vi "WebDAV address (global).vi"(0 "Network Drive IP":string, 1 "Mode":enum16{"Read", "Write"}(ring)) -> (2 "WebDAV Address":string)   [LabVIEW 2013]
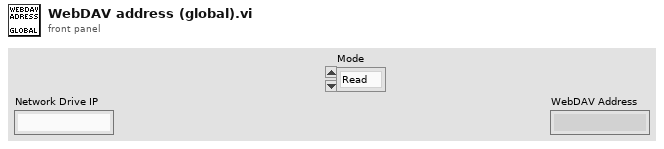
[diagram p1: front panel]
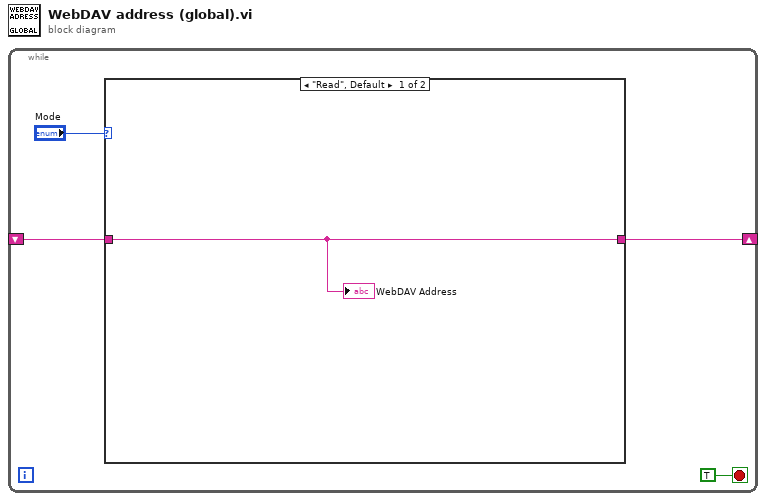
[diagram p0: block diagram]
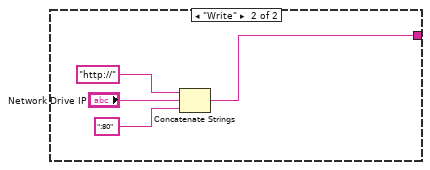
[diagram p2: hidden frame]
diagram:
  n1 = while {
    shift-right: [w2] -> _
    shift-left: _ -> [w1]
    stop <- TRUE stop-if-true
    n2 = case shown="\"Read\", Default" "Mode" {
      tunnel: [w5 w6] -> w2
      tunnel: w1 -> [w5 _]
      frame "Read", Default {
        "WebDAV Address" <- w5
      }
      frame "Write" {
        n3 = Concatenate Strings("http://", "Network Drive IP", ":80") -> (w6:string)
      }
    }
  }
